vi "Validate Subsystems.vi"(8 "error in (no error)":errorcluster, 10 "UI Message Queue In":refnum<queue>, 11 "System Configuration":T1) -> (0 "error out":errorcluster, 2 "UI Message Queue Out":refnum<queue>, 3 "dup System Configuration":T1)   [LabVIEW 2024]
doc: "Validates all the subsystems and updates log to report a warning when the source binding URL is invalid."
uses:
  Controls/Server/System Configuration.ctl
  Controls/Server/Subsystem Configuration.ctl
  Shared/Message Queue/Message Cluster.ctl
  Shared/Message Queue.lvlib
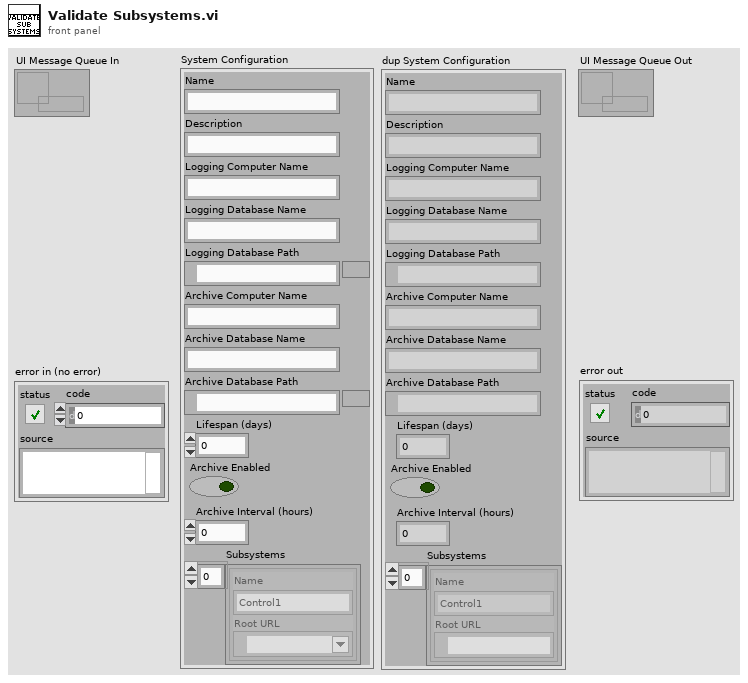
[diagram p1: front panel]
types:
  T1 = typedef "System Configuration.ctl" = cluster{"Name":string, "Description":string, "Logging Computer Name":string, "Logging Database Name":string, "Logging Database Path":path, "Archive Computer Name":string, "Archive Database Name":string, "Archive Database Path":path, "Lifespan (days)":u32, "Archive Enabled":bool, "Archive Interval (hours)":u32, "Subsystems":T2[]}
  T2 = typedef "Subsystem Configuration.ctl" = cluster{"Name":string, "Root URL":refnum<k21>}
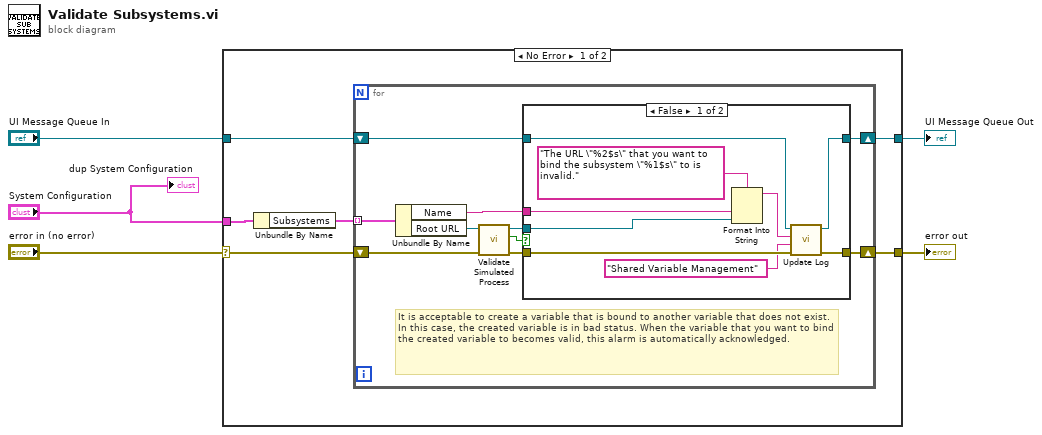
[diagram p0: block diagram]
diagram:
  n1 = case shown="No Error" "error in (no error)" {
    selector: "error in (no error)" -> [w7 w34]
    tunnel: [w8 w34] -> w4
    tunnel: "System Configuration" -> [w10 _]
    tunnel: "UI Message Queue In" -> [w6 w33]
    tunnel: [w9 w33] -> w1
    frame No Error {
      n2 = Unbundle By Name(w10) -> ("Subsystems"=w11:T2[])
      n3 = for {
        tunnel: w11 -> [w20] mode=indexing
        shift-right: [w14] -> w9
        shift-left: w6 -> [w12]
        shift-right: [w21] -> w8
        shift-left: w7 -> [w13]
        # "It is acceptable to create a variable that is bound to another variable that does not exist. In this case, the created variable is in bad status. When the variable that you want to bind the created variable to becomes valid, this alarm is automatically acknowledged."
        n4 = Unbundle By Name(w20) -> ("Name"=w16:string, "Root URL"=w18:refnum<k21>)
        n5 = call "Validate Simulated Process.vi"("error in (no error)"=w13, "URL"=w18) -> ("error out"=w19:errorcluster, "Valid?"=w17:bool, "dup URL"=w15:refnum<k21>)  [unwired: 7 in]
        n6 = case shown="False" w17 {
          tunnel: [w30 w32] -> w21
          tunnel: w19 -> [w29 w32]
          tunnel: w12 -> [w28 w31]
          tunnel: w16 -> [w25 _]
          tunnel: w15 -> [w24 _]
          tunnel: [w22 w31] -> w14
          frame False {
            n7 = Format Into String(format string="The URL \"%2$s\" that you want to bind the subsystem \"%1$s\" to is invalid." ("Component"), w25, w24) -> (resulting string=w23:string)  [unwired: 2 in, 1 out]
            n8 = call "Update Log.vi"("error in (no error)"=w29, "Component"="Shared Variable Management", "Status"=w23, "UI Message Queue"=w28) -> ("error out"=w30:errorcluster, "dup UI Message Queue"=w22:refnum<queue>)  [unwired: 5 in, 1 out]
          }
          frame True {
          }
        }
      }
    }
    frame Error {
    }
  }
  "error out" <- w4
  "UI Message Queue Out" <- w1
  "dup System Configuration" <- "System Configuration"
